vi "Acquire Analyze Visualize - Part 2.vi"() -> ()   [LabVIEW 2020]
uses:
  <vilib>/DAQmx/read.llb/DAQmx Read (Analog DBL 1Chan 1Samp).vi
  <vilib>/DAQmx/miscellaneous.llb/DAQmx Fill In Error Info.vi
panel:
  out "Message":string
  out "Threshold Exceeded?":bool
  in  "Maximum Threshold (deg C)":dbl(slide)=30.0 min=15.0 max=50.0 step=1.0 scale=15.0..50.0
  out "Current Temperature (deg C)":dbl
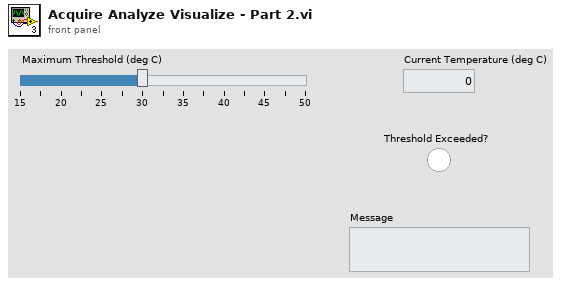
[diagram p1: front panel]
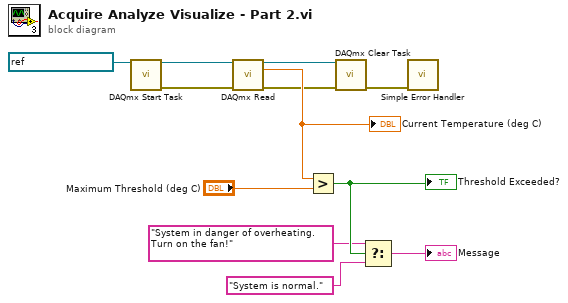
[diagram p0: block diagram]
diagram:
  n1 = call <vilib>:"DAQmx Start Task.vi"("task/channels in"=refnum<k21> "Thermocouple" ("DAQmx Task Name")) -> ("task out"=w5:refnum<k21>, "error out"=w7:errorcluster)  [unwired: 13 in]
  n2 = call-poly <vilib>:"DAQmx Read.vi"("task/channels in"=w5, "error in"=w7) -> ("task out"=w6:refnum<k21>, "data"=w9:dbl, "error out"=w8:errorcluster)  [unwired: 11 in]
  "Current Temperature (deg C)" <- w9
  n3 = Greater?(x=w9, y="Maximum Threshold (deg C)") -> (0:w12:bool)
  "Threshold Exceeded?" <- w12
  n4 = call <vilib>:"DAQmx Clear Task.vi"("task in"=w6, "error in"=w8) -> ("error out"=w1:errorcluster)  [unwired: 13 in]
  n5 = Select(t="System in danger of overheating. Turn on the fan!", s=w12, f="System is normal.") -> (s? t:f=→"Message":string)
  n6 = call <vilib>:"Simple Error Handler.vi"("error in (no error)"=w1) -> ()  [unwired: 4 in, 5 out]
